vi "插入数据.vi"(5 "data":variant, 7 "columns":string[](array[string]), 8 "error in (no error)":errorcluster, 10 "database":string, 11 "table":string) -> (0 "error out":errorcluster)   [LabVIEW 2016, in "数据传输系统-03.lvlib"]
uses:
  <vilib>/Utility/sysdir.llb/System Directory Type.ctl
  <vilib>/addons/database/Connection.llb/DB Tools Open Connec (String).vi
  <vilib>/addons/database/NI_Database_API.lvlib
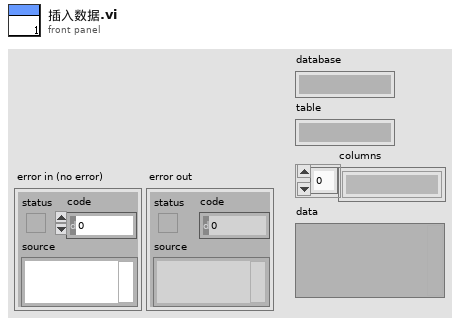
[diagram p1: front panel]
types:
  T1 = typedef "System Directory Type.ctl" = i32
  T2 = typedef "NI_Database_API.lvlib/Conn ObjectReference.ctl" = refnum<k1>
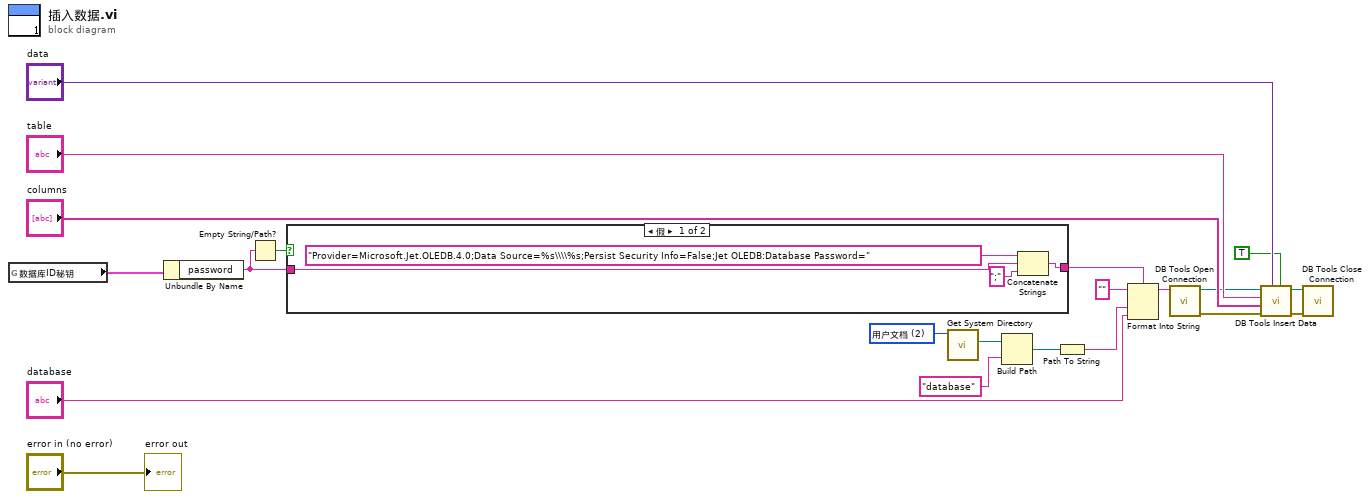
[diagram p0: block diagram]
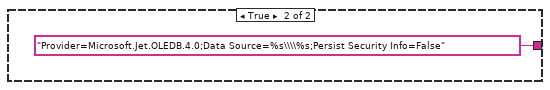
[diagram p2: hidden frame]
diagram:
  w16 = T1 2 items=["用户目录"=0, "用户桌面"=1, "用户文档"=2, "用户应用程序数据"=3, "用户设置"=4, "用户临时目录"=5, "公共文档"=6, "公共应用程序数据"=7, "公共设置"=8, "公共缓存"=13, "系统核心库"=9, "系统安装库"=10, "应用程序文件"=11, "启动盘根目录"=12] ("system directory type")
  n1 = global read "外部交互全局.vi" "数据库ID秘钥"() -> (w1:cluster{"userID":string, "password":string})
  n2 = Unbundle By Name(w1) -> ("password"=w8:string)
  n3 = Empty String/Path?(string/path=w8) -> (empty?=w9:bool)
  n4 = case shown="假" w9 {
    tunnel: [w22 "Provider=Microsoft.Jet.OLEDB.4.0;Data Source=%s\\\\%s;Persist Security Info=False" ("格式字符串")] -> w6
    tunnel: w8 -> [w25 _]
    frame False {
      n5 = Concatenate Strings("Provider=Microsoft.Jet.OLEDB.4.0;Data Source=%s\\\\%s;Persist Security Info=False;Jet OLEDB:Database Password=" ("格式字符串"), w25, ";" ("字符串")) -> (w22:string)
    }
    frame True {
    }
  }
  n6 = call <vilib>:"Get System Directory.vi"("system directory type"=w16) -> ("system directory"=w15:path)  [unwired: 10 in]
  n7 = Build Path(base path=w15, name or relative path="database" ("condition")) -> (appended path=w14:path)
  n8 = Path To String(path=w14) -> (string=w4:string)
  n9 = Format Into String(format string=w6, initial string="" ("初始字符串"), w4, "database") -> (resulting string=w5:string)  [unwired: 1 in, 1 out]
  n10 = call-poly <vilib>:"DB Tools Open Connection.vi"("connection information"=w5) -> ("error out"=w11:errorcluster, "connection reference"=w12:T2)  [unwired: 7 in]
  n11 = call <vilib>:"DB Tools Insert Data.vi"("create table? (F)"=TRUE, "data"="data", "error in (no error)"=w11, "columns"="columns", "table"="table", "connection reference"=w12) -> ("error out"=w20:errorcluster, "connection reference out"=w21:T2)  [unwired: 4 in]
  n12 = call <vilib>:"DB Tools Close Connection.vi"("error in (no error)"=w20, "connection reference"=w21) -> ()  [unwired: 5 in, 1 out]
  "error out" <- "error in (no error)"
